vi "STORAGE.vi"() -> (0 "High Bank Pressure":dbl, 1 "Medium Bank Pressure":dbl, 2 "Low Bank Pressure":dbl, 3 "HB Trend":i32(graph), 4 "MB Trend":i32(graph), 5 "LB Trend":i32(graph))   [LabVIEW 2014]
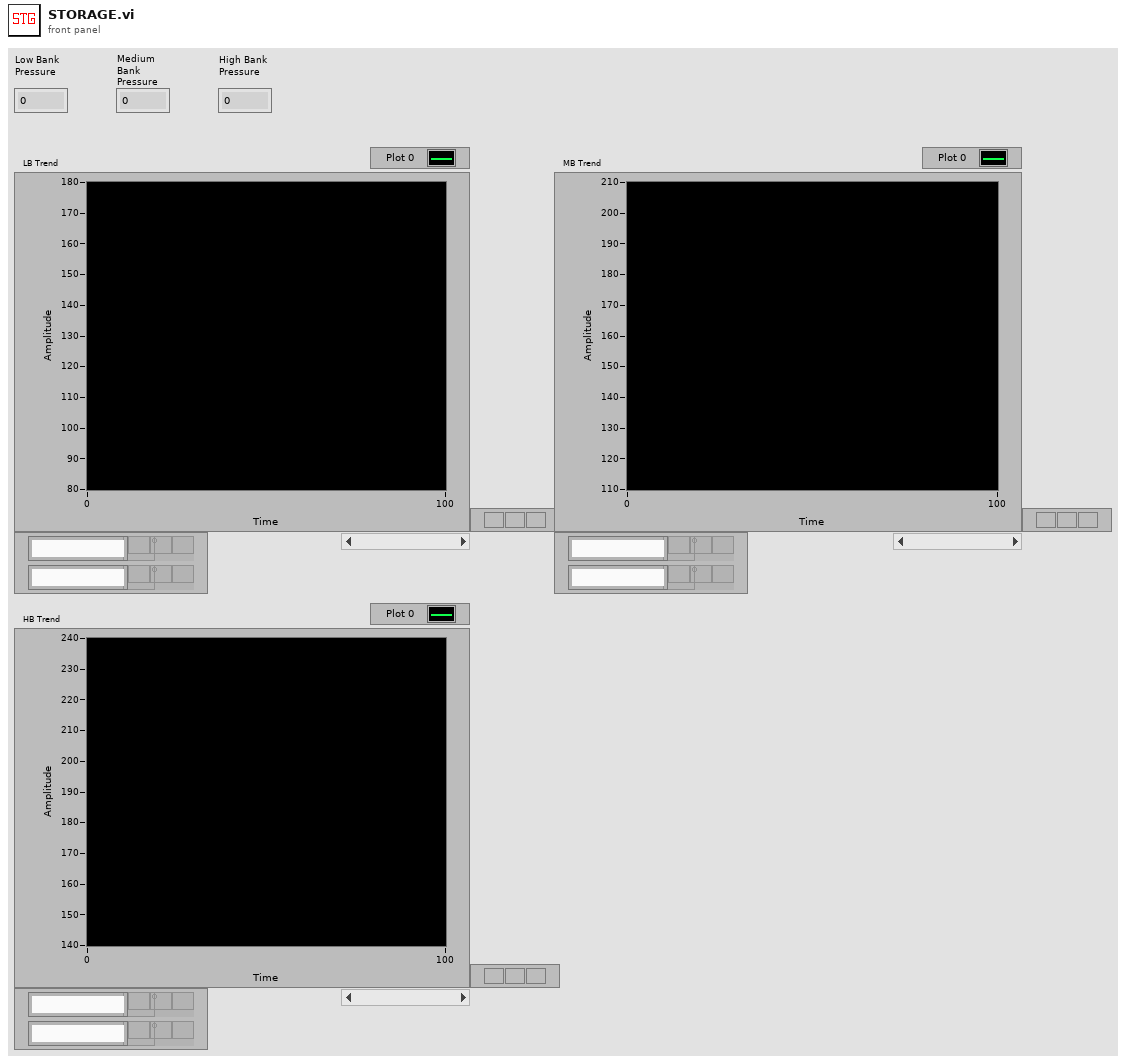
[diagram p1: front panel]
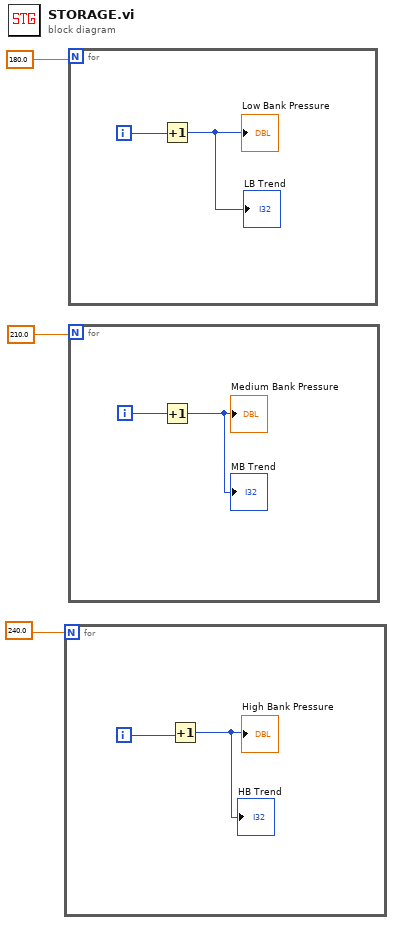
[diagram p0: block diagram]
diagram:
  n1 = for {
    N: 240.0 -> [_]
    i -> [w5]
    n2 = Increment(x=w5) -> (x+1=→"High Bank Pressure" →"HB Trend":i32)
  }
  n3 = for {
    N: 180.0 -> [_]
    i -> [w7]
    n4 = Increment(x=w7) -> (x+1=→"Low Bank Pressure" →"LB Trend":i32)
  }
  n5 = for {
    N: 210.0 -> [_]
    i -> [w9]
    n6 = Increment(x=w9) -> (x+1=→"Medium Bank Pressure" →"MB Trend":i32)
  }
